vi "POST Multipart.vi"(0 "client handle":T5, 1 "output file":path=path "", 2 "Error code options":T2={"1xx (info)"=FALSE, "2xx (success)"=FALSE, "3xx (redirect)"=FALSE, "4xx (client error)"=TRUE, "5xx (server error)"=TRUE, "Other"=TRUE}, 3 "BlueLogParent in":refnum<class "BlueLogParent_OpenSource.lvclass">, 5 "url":string, 7 "data":T3[](array[typedef]), 11 "error in (no error)":errorcluster, 12 "timeout (10000)":i32=10000) -> (4 "client handle out":T5, 6 "headers":T4[](array[typedef]), 8 "body":string, 10 "HTTP response code":T1, 15 "error out":errorcluster)   [LabVIEW 2020, in "Blue Easy HTTP OpenSource.lvlib"]
doc: "Sends a Web request that submits multiple sets of data or files to a server, Web page, or Web service. This VI uses the POST HTTP method and multipart/form-data MIME type. Refer to the World Wide Web Consortium Web site at www.w3.org for more information about the POST method and the multipart content type.\n\nThe POSTMultipart VI submits multiple sets of data, represented by an array of postdata clusters. The POSTMultipart VI determines which data format to accept from the client and which format to send the data to the server based upon the controls specified within each postdata cluster. Use the postdata control descriptions to configure the submitted data as one of the four available combinations. For example, the VI can accept a buffer data string from the client and send that data as a file to the server."
uses:
  Blue Easy HTTP OpenSource.lvlib
  <vilib>/httpClient/ClientHandle.ctl
  HTTP Header.ctl
  <vilib>/httpClient/MultipartData.ctl
  HTTP error on codes.ctl
  HTTP response code.ctl
  <userlib>/Blue Origin/BlueLogParent_OpenSource/BlueLogParentClass/BlueLogParent_OpenSource.lvclass
  Interpret Header.vi
  <vilib>/dlg_ctls.llb/Space Constant.vi
  <vilib>/Utility/error.llb/Trim Whitespace.vi
  <vilib>/Utility/error.llb/Error Cluster From Error Code.vi
  <vilib>/httpClient/LabVIEWHTTPClient.lvlib
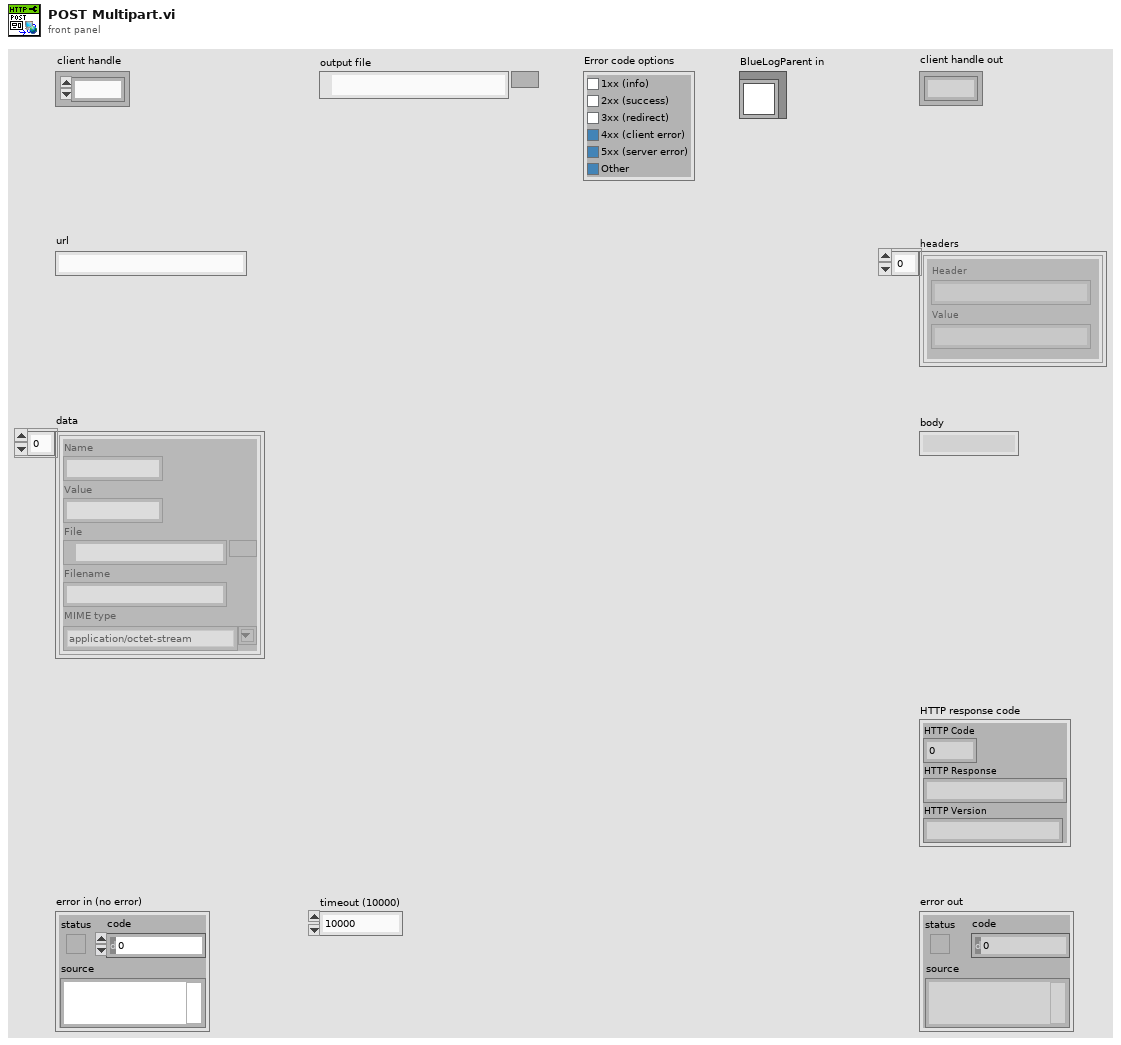
[diagram p1: front panel]
types:
  T1 = typedef "Blue Easy HTTP OpenSource.lvlib/HTTP response code.ctl" = cluster{"HTTP Code":u16, "HTTP Response":string, "HTTP Version":string}
  T2 = typedef "Blue Easy HTTP OpenSource.lvlib/HTTP error on codes.ctl" = cluster{"1xx (info)":bool, "2xx (success)":bool, "3xx (redirect)":bool, "4xx (client error)":bool, "5xx (server error)":bool, "Other":bool}
  T3 = typedef "LabVIEWHTTPClient.lvlib/MultipartData.ctl" = cluster{"Name":string, "Value":string, "File":path, "Filename":string, "MIME type":string}
  T4 = typedef "Blue Easy HTTP OpenSource.lvlib/HTTP Header.ctl" = cluster{"Header":string, "Value":string}
  T5 = typedef "LabVIEWHTTPClient.lvlib/ClientHandle.ctl" = refnum<k1>
  T6 = typedef "BlueLogParent_OpenSource.lvclass/BlueLogParentLevel.ctl" = enum16{"DEBUG", "INFO", "WARNING", "ERROR", "CRITICAL"}
  T7 = typedef "BlueLogParent_OpenSource.lvclass/BlueLogParentOptions.ctl" = cluster{"timestamp (now)":dbl, "Call chain (here)":string, "Count (1)":u16, "Font (override)":T8, "Add row separator? (T)":bool}
  T8 = typedef "BlueLogParent_OpenSource.lvclass/BlueLogParentFont.ctl" = cluster{"Font Name":string, "Size":u16, "Bold":bool, "Italic":bool, "Underline":bool, "Strikeout":bool, "Color":u32}
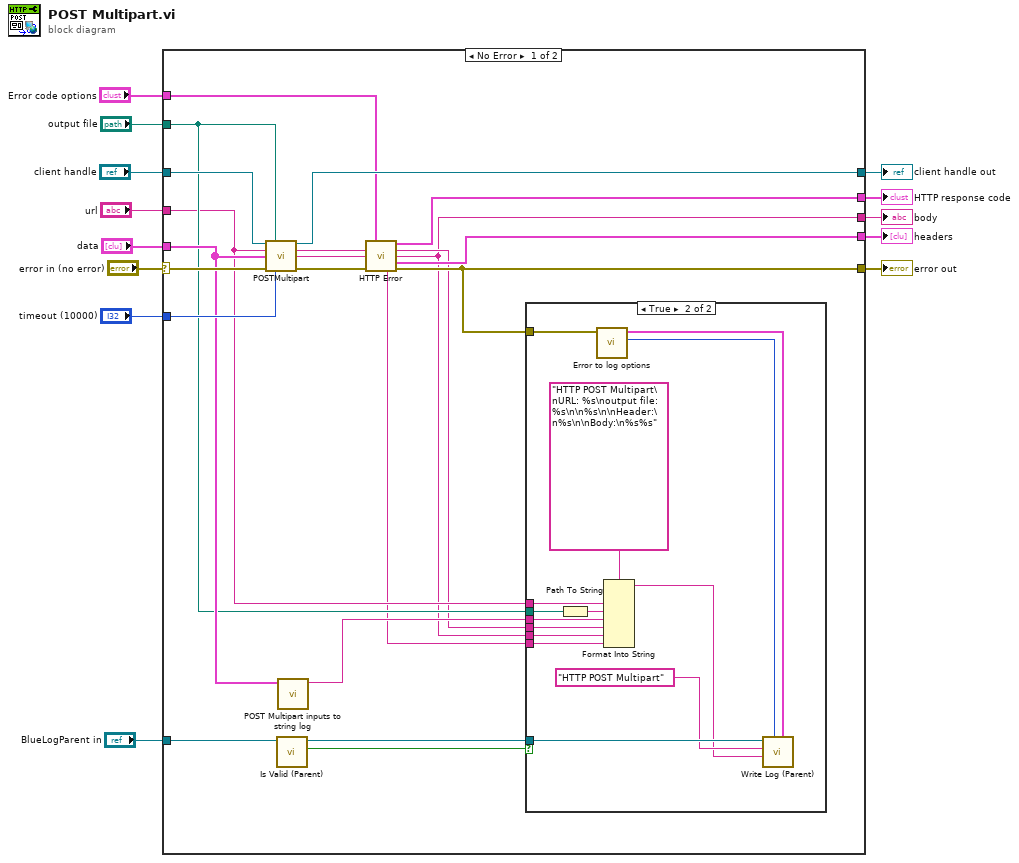
[diagram p0: block diagram]
diagram:
  n1 = case shown="No Error" "error in (no error)" {
    selector: "error in (no error)" -> [w34 w50]
    tunnel: [w25 w50] -> w13
    tunnel: "timeout (10000)" -> [w33 _]
    tunnel: "data" -> [w26 _]
    tunnel: "url" -> [w23 _]
    tunnel: "client handle" -> [w32 w49]
    tunnel: "output file" -> [w24 _]
    tunnel: [w31 w49] -> w6
    tunnel: [w27 _] -> w5
    tunnel: "Error code options" -> [w29 _]
    tunnel: [w28 _] -> w3
    tunnel: [w15 _] -> w2
    tunnel: "BlueLogParent in" -> [w19 _]
    frame No Error {
      n2 = call <vilib>:"POSTMultipart.vi"("client handle"=w32, "output file"=w24, "url"=w23, "data"=w26, "error in (no error)"=w34, "timeout (10000)"=w33) -> ("client handle out"=w31:T5, "headers"=w21:string, "body"=w20:string, "error out"=w30:errorcluster)  [unwired: 6 in]
      n3 = call-dynamic "Is Valid (Parent).vi"("BlueLogParent in"=w19) -> ("Is Valid?"=w18:bool, "BlueLogParent out"=w17:refnum<class "BlueLogParent_OpenSource.lvclass">)  [unwired: 8 in, 1 out]
      n4 = call "POST Multipart inputs to string log.vi"("POST inputs"=w26) -> ("POST inputs"=w22:string)  [unwired: 10 in]
      n5 = call "HTTP Error.vi"("Error code options"=w29, "Header"=w21, "body"=w20, "error in (no error)"=w30) -> ("HTTP response code"=w28:T1, "Header (dup)"=w16:string, "body (dup)"=w15:string, "Header Values"=w27:T4[], "Error log"=w14:string, "error out"=w25:errorcluster)  [unwired: 6 in]
      n6 = case shown="True" w18 {
        tunnel: w25 -> [_ w40]
        tunnel: w23 -> [_ w47]
        tunnel: w24 -> [_ w46]
        tunnel: w22 -> [_ w44]
        tunnel: w15 -> [_ w43]
        tunnel: w16 -> [_ w42]
        tunnel: w17 -> [_ w41]
        tunnel: w14 -> [_ w35]
        frame False {
        }
        frame True {
          n7 = Path To String(path=w46) -> (string=w45:string)
          n8 = call "Error to log options.vi"("error in (no error)"=w40) -> ("Logging level"=w39:T6, "Options"=w38:T7)  [unwired: 9 in]
          n9 = Format Into String(format string="HTTP POST Multipart\nURL: %s\noutput file: %s\n\n%s\n\nHeader:\n%s\n\nBody:\n%s%s", w47, w45, w44, w42, w43, w35) -> (resulting string=w36:string)  [unwired: 2 in, 1 out]
          n10 = call-dynamic "Write Log (Parent).vi"("Options"=w38, "Logging level (INFO)"=w39, "Message"=w36, "Message Title"="HTTP POST Multipart" ("Unique ID"), "BlueLogParent in"=w41) -> ()  [unwired: 5 in, 2 out]
        }
      }
    }
    frame Error {
    }
  }
  "error out" <- w13
  "client handle out" <- w6
  "headers" <- w5
  "HTTP response code" <- w3
  "body" <- w2
